vi "Msg.vi"(7 "LVCAM in":refnum<class "LVCAM.lvclass">, 11 "Msg in":refnum<class "Msg.lvclass">) -> (0 "error out":errorcluster, 2 "Destroyed Self?":bool, 5 "LVCAM out":refnum<class "LVCAM.lvclass">)   [LabVIEW 2021, in "LVCAM.lvlib" / "Msg.lvclass"]
uses:
  Msg.lvclass
  LVCAM/LVCAM.lvclass
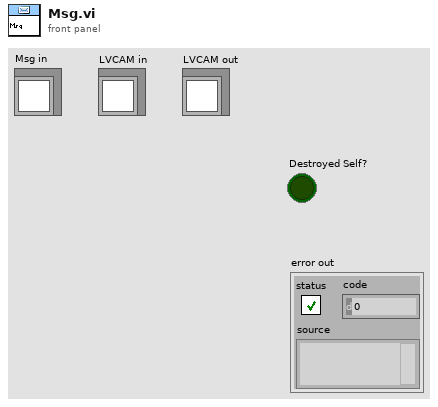
[diagram p1: front panel]
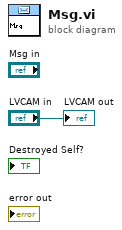
[diagram p0: block diagram]
diagram:
  "LVCAM out" <- "LVCAM in"
